vi "copyLog.vi"(8 "error in (no error)":errorcluster, 11 "Text reference":refnum<vi>) -> (0 "error out":errorcluster)   [LabVIEW 2017]
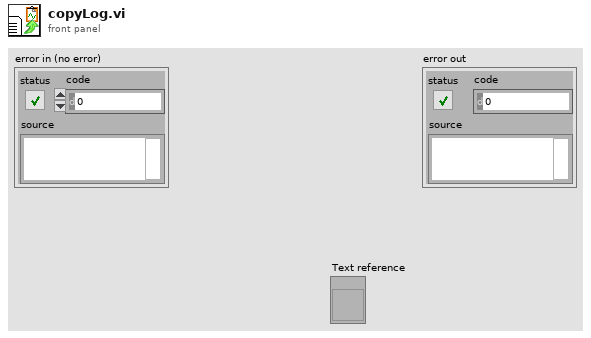
[diagram p1: front panel]
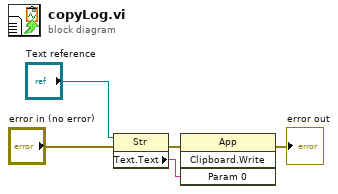
[diagram p0: block diagram]
diagram:
  n1 = property class="Str"(reference="Text reference", error in="error in (no error)") -> (error out=w3:errorcluster, "Text.Text"=w4:string)  [unwired: 1 out]
  n2 = invoke class="App" method="Clipboard.Write"(error in=w3, "Param 0"=w4) -> (error out=→"error out":errorcluster)  [unwired: 2 in, 3 out]
